vi "applicationStart.vi"(8 "error in":errorcluster, 10 "File Path":path, 11 "controlsArray":refnum<vi>[](array[refnum])) -> (0 "error out":errorcluster, 3 "fileRef":refnum<file>)   [LabVIEW 2024]
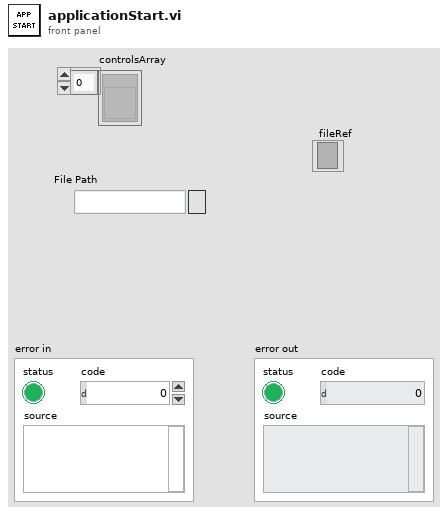
[diagram p1: front panel]
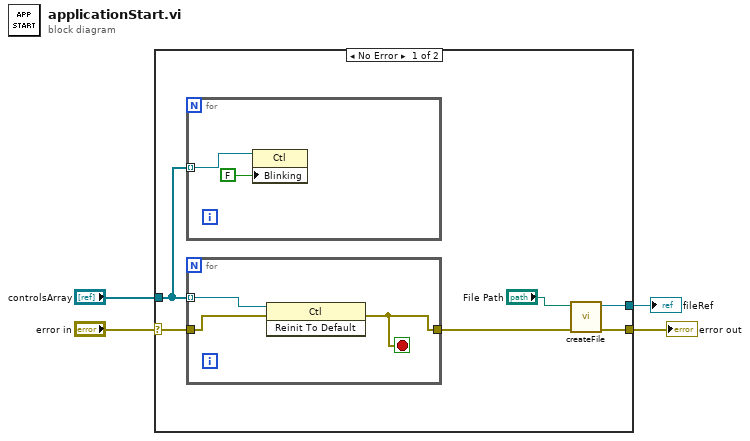
[diagram p0: block diagram]
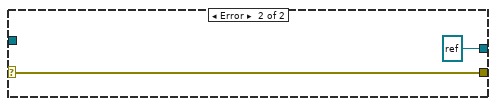
[diagram p2: hidden frame]
diagram:
  n1 = case shown="No Error" "error in" {
    selector: "error in" -> [w10 w17]
    tunnel: [w8 w17] -> w3
    tunnel: "controlsArray" -> [w5 _]
    tunnel: [w6 refnum<file> refnum ("fileRef")] -> w1
    frame No Error {
      n2 = for {
        tunnel: w5 -> [w12] mode=indexing
        n3 = property class="Ctl"(reference=w12, "Blinking"=FALSE) -> ()  [unwired: 1 in, 2 out]
      }
      n4 = for {
        tunnel: w5 -> [w15] mode=indexing
        tunnel: w10 -> [w14]
        tunnel: [w13] -> w9
        stop <- w13 stop-if-true
        n5 = invoke class="Ctl" method="Reinit To Default"(reference=w15, error in=w14) -> (error out=w13:errorcluster)  [unwired: 1 in, 2 out]
      }
      n6 = call "createFile.vi"("error in"=w9, "File Path"="File Path") -> ("error out"=w8:errorcluster, "fileRef"=w6:refnum<file>)  [unwired: 8 in]
    }
    frame Error {
    }
  }
  "error out" <- w3
  "fileRef" <- w1
